vi "StopProcess_SET.vi"(8 "error in":errorcluster, 10 "notification":bool, 11 "lia host in":refnum<class "LIA Host Interface RT.lvclass">) -> (0 "error out":errorcluster, 3 "lia host out":refnum<class "LIA Host Interface RT.lvclass">)   [LabVIEW 2018, in "LIA Host Interface RT.lvclass"]
uses:
  LIA Host Interface RT.lvclass
  LIA Host Interface RT.lvclass/LIA Host Interface RT.ctl
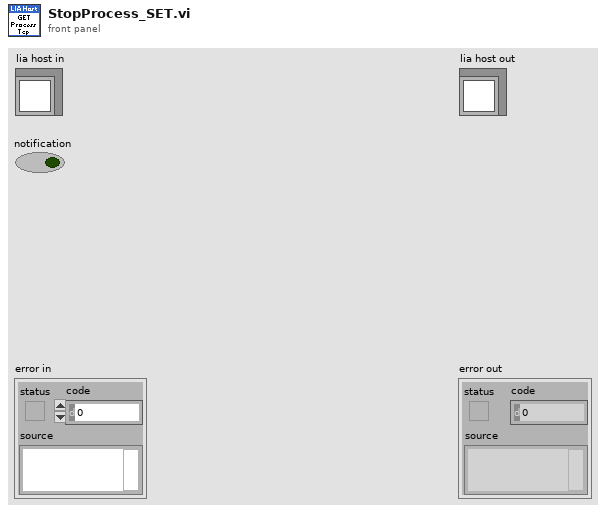
[diagram p1: front panel]
types:
  T1 = typedef "Lock-In Amplifier Host RT.lvclass/session data.ctl" = cluster{"tcp connection":refnum<k5>, "incoming data":refnum<queue>, "outgoing data":refnum<queue>, "lock-in data":refnum<queue>[], "stop process":refnum<notifier>}
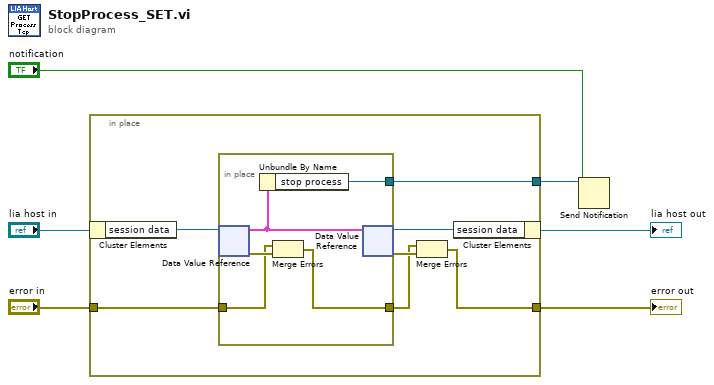
[diagram p0: block diagram]
diagram:
  n1 = in-place {
    in-place-border: [w11] -> w2
    in-place-border: "error in" -> [w10]
    in-place-border: [w7] -> w3
    n2 = in-place-cluster #1("lia host in") -> ("session data"=w13:refnum<data-value>)
    n3 = in-place {
      in-place-border: [w17] -> w11
      in-place-border: w10 -> [w15]
      in-place-border: [w14] -> w8
      n4 = in-place-dvr #2(w13) -> (w18:T1, w16:errorcluster)
      n5 = Unbundle By Name(w18) -> ("stop process"=w17:refnum<notifier>)
      n6 = Merge Errors(w15, w16) -> (w14:errorcluster)
      n7 = in-place-dvr #2(w18) -> (w12:refnum<data-value>, w9:errorcluster)
    }
    n8 = Merge Errors(w8, w9) -> (w7:errorcluster)
    n9 = in-place-cluster #1("session data"=w12) -> (→"lia host out":refnum<class "LIA Host Interface RT.lvclass">)
  }
  "error out" <- w3
  n10 = Send Notification(notification="notification", notifier=w2) -> ()  [unwired: 1 in, 2 out]
